vi "Runtime Test.vi"() -> (0 "final error":errorcluster, 1 "correct execution settings":bool, 3 "Pass":bool)   [LabVIEW 2015, in "SystemLink File Module tests.lvlib"]
doc: "This VI shows an example for how to test the Runtime functionality of the module. This will need to be modified according to module functionality."
uses:
  SystemLink File Module tests.lvlib
  module/execution/SystemLink File runtime.lvclass
  <vilib>/NI/Tag Bus/dictionary/data dictionary.lvclass/data dictionary.ctl
  <vilib>/NI/Tag Bus/dictionary/lookup polymorphs/locate Boolean.vi
  <vilib>/NI/Tag Bus/table/data polymorphs/write one/write Boolean.vi
  <vilib>/NI/Tag Bus/dictionary/search/find data index.vi
  <vilib>/NI/Tag Bus/dictionary/search/search string list.vi
  <vilib>/Skyline/File/Filter/Create Filter (Name).vi
  <vilib>/NI/Tag Bus/dictionary/tag not found.vi
  module/configuration/SystemLink File configuration.lvclass
  <vilib>/NI/Tag Bus/dictionary/data dictionary.lvclass
  <vilib>/NI/Tag Bus/table/data table.lvlib
  <vilib>/Skyline/File/File/NI Skyline File.lvclass
  <vilib>/Skyline/File/Filter/NI Skyline File Filter.lvclass
panel:
  out "Names":string[](array[string])
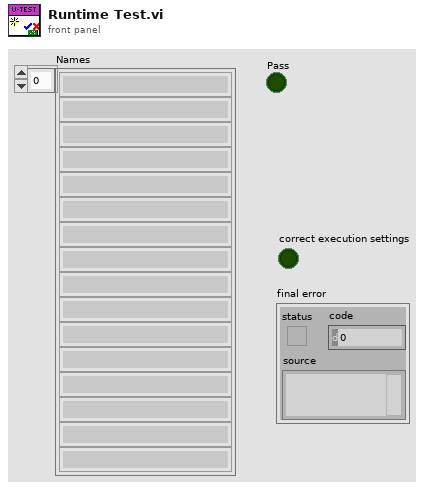
[diagram p1: front panel]
types:
  T1 = typedef "TBM channel.lvclass/data tables.ctl" = cluster{"input data":T2, "processing parameter":T2, "processing result":T2, "output data":T2}
  T2 = typedef "tag bus.lvlib/dictionary table pair.ctl" = cluster{"data dictionary":refnum<class "data dictionary.lvclass">, "data table":T3}
  T3 = typedef "tag bus.lvlib/data table.lvlib/data table.ctl" = cluster{"Double":dbl[], "Single":sgl[], "I64":i64[], "I32":i32[], "I16":i16[], "I8":i8[], "U64":u64[], "U32":u32[], "U16":u16[], "U8":u8[], "Boolean":bool[], "String":string[], "Array of Double":cluster{"DBL Array":dbl[]}[], "Array of Single":cluster{"SGL Array":sgl[]}[], "Array of I64":cluster{"I64 Array":i64[]}[], "Array of I32":cluster{"I32 Array":i32[]}[], "Array of I16":cluster{"I16 Array":i16[]}[], "Array of I8":cluster{"I8 Array":i8[]}[], "Array of U64":cluster{"U64 Array":u64[]}[], "Array of U32":cluster{"U32 Array":u32[]}[], "Array of U16":cluster{"U16 Array":u16[]}[], "Array of U8":cluster{"U8 Array":u8[]}[], "Array of Boolean":cluster{"Boolean Array":bool[]}[], "Array of String":cluster{"String Array":string[]}[]}
  T4 = typedef "TBM module execution interface.lvclass/execution settings.ctl" = cluster{"reads inputs":bool, "processes data":bool, "writes outputs":bool}
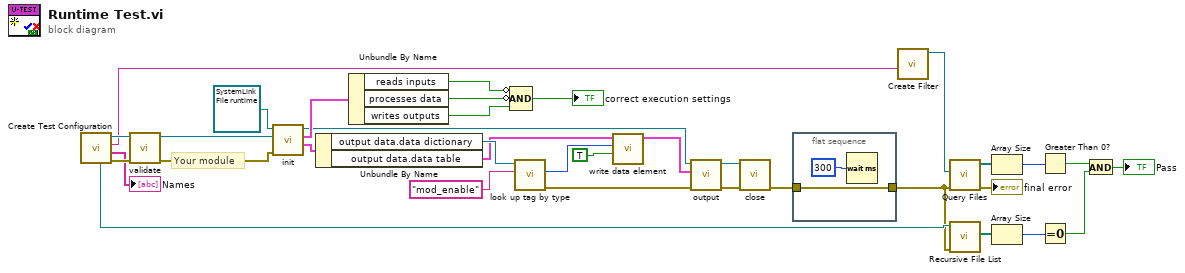
[diagram p0: block diagram]
diagram:
  # "Your module"
  n1 = call "Create Test Configuration.vi"() -> ("error out"=w25:errorcluster, "Names"=→"Names":string[], "File Name"=w12:string, "Module Configuration"=w26:refnum<class "SystemLink File configuration.lvclass">, "Folder Path"=w7:path)  [unwired: 5 in, 2 out]
  n2 = call-dynamic "validate.vi"("error in"=w25, "SystemLin Tag Module configuration in"=w26) -> ("error out"=w34:errorcluster, "SystemLin Tag Module configuration out"=w35:refnum<class "SystemLink File configuration.lvclass">)  [unwired: 8 in]
  n3 = call-dynamic "init.vi"("error in"=w34, "TBM module configuration in"=w35, "SystemLin Tag Module runtime in"=refnum<class "SystemLink File runtime.lvclass"> refnum ("tag bus configurable plugin module")) -> ("data allocations"=w27:T1, "execution settings"=w32:T4, "SystemLin Tag Module runtime out"=w23:refnum<class "SystemLink File runtime.lvclass">)  [unwired: 5 in, 1 out]
  n4 = Unbundle By Name(w27) -> ("output data.data dictionary"=w21:refnum<class "data dictionary.lvclass">, "output data.data table"=w17:T3)
  n5 = Unbundle By Name(w32) -> ("reads inputs"=w29:bool, "processes data"=w31:bool, "writes outputs"=w30:bool)
  n6 = Compound Arithmetic op=AND(invert w29, invert w31, w30) -> (→"correct execution settings":bool)
  n7 = call-poly <vilib>:"look up tag by type.vi"("name"="mod_enable" ("channel name"), "data dictionary in"=w21) -> ("error out"=w15:errorcluster, "index"=w19:i32)  [unwired: 7 in, 1 out]
  n8 = call-poly <vilib>:"write data element.vi"("value"=TRUE, "index"=w19, "data table in"=w17) -> ("data table out"=w16:T3)  [unwired: 8 in]
  n9 = call-dynamic "output.vi"("error in"=w15, "data table in"=w16, "SystemLin Tag Module runtime in"=w23) -> ("error out"=w14:errorcluster, "SystemLin Tag Module runtime out"=w22:refnum<class "SystemLink File runtime.lvclass">)  [unwired: 6 in, 1 out]
  n10 = call-dynamic "close.vi"("error in"=w14, "SystemLin Tag Module runtime in"=w22) -> ("error out"=w9:errorcluster)  [unwired: 9 in]
  n11 = flat-sequence {
    tunnel: [w36] -> w1
    tunnel: w9 -> [w36]
    frame #0 {
      n12 = Wait (ms)(milliseconds to wait=u32 300) -> ()  [unwired: 1 out]
    }
  }
  n13 = call-poly <vilib>:"Create Filter.vi"("value"=w12) -> ("filter out"=w13:refnum<class "NI Skyline File Filter.lvclass">)  [unwired: 9 in, 1 out]
  n14 = call <vilib>:"Query Files.vi"("error in (no error)"=w1, "filter"=w13) -> ("error out"=→"final error":errorcluster, "available files"=w11:refnum<class "NI Skyline File.lvclass">[])  [unwired: 7 in, 1 out]
  n15 = call <vilib>:"Recursive File List.vi"("error in (no error)"=w1, "Folder Path"=w7) -> ("All Files in Dir"=w6:path[])  [unwired: 5 in, 4 out]
  n16 = Array Size(array=w11) -> (size(s)=w10:i32)
  n17 = Array Size(array=w6) -> (size(s)=w5:i32)
  n18 = Greater Than 0?(x=w10) -> (x > 0?=w3:bool)
  n19 = Equal To 0?(x=w5) -> (x = 0?=w4:bool)
  n20 = And(x=w3, y=w4) -> (x .and. y?=→"Pass":bool)
